vi "Stim_control_v17.vi"() -> ()   [LabVIEW 2010]
doc: "Use this template to measure or generate signals using the DAQ Assistant Express VI and NI-DAQmx. Double click the DAQ Assistant Express VI to launch a configuration wizard which steps you through configuring a measurement or generation.\n\nNote: You must have an NI-DAQmx compatible device installed to use this Express VI. Refer to the DAQ Quick Start Guide for NI-DAQ 7.0 for a list of compatible devices."
uses:
  <vilib>/Analysis/3filter.llb/Filter Passband Type.ctl
  <vilib>/DAQmx/write.llb/DAQmx Write (Digital Bool 1Line 1Point).vi
  <vilib>/DAQmx/write.llb/DAQmx Write (Analog 1D DBL 1Chan NSamp).vi
  <vilib>/DAQmx/read.llb/DAQmx Read (Analog 2D I16 NChan NSamp).vi
  <vilib>/daqmx/miscellaneous.llb/DAQmx Fill In Error Info.vi
  <vilib>/Utility/file.llb/Write To Spreadsheet File (DBL).vi
  <vilib>/DAQmx/create/channels.llb/DAQmx Create Channel (DO-Digital Output).vi
  <vilib>/DAQmx/create/channels.llb/DAQmx Create Channel (AO-Voltage-Basic).vi
  <vilib>/DAQmx/configure/timing.llb/DAQmx Timing (Sample Clock).vi
  <vilib>/DAQmx/configure/trigger.llb/DAQmx Start Trigger (Digital Edge).vi
  <vilib>/DAQmx/create/channels.llb/DAQmx Create Channel (AI-Voltage-Basic).vi
  Program Files/National Instruments/LabVIEW 2010/resource/objmgr/daqmx.rc
  <vilib>/Analysis/NI_AALBase.lvlib
  <vilib>/ptbypt/NI_PtbyPt.lvlib
panel:
  in  "ms to check for trigger":u32=5
  out "within file Datapoint number":u32
  out "Datapoint number":u32
  out "Detect On":bool
  out "Packet Size":i32
  in  "Stims before saving new file":dbl=200.0
  out "stimtrain_savename":path
  out "Stim rate":dbl
  out "Stim train loaded?":bool
  out "N Files":u32=1
  in  "Output Data Root":path=path "C:/DATA/gr15lb165"
  out "Current File":path
  in  "Bird Name":string="gr15lb165_250uA_2pulses"
  in  "File Open?":bool
  out "Outfile RefNum":refnum<file>
  out "Catch?":bool
  out "stim train number":u32
  out "Reset Trig Error 2":errorcluster
  in  "Manual Trigger":bool
  in  "calibration On?":bool
  out "AI Error":errorcluster
  in  "Data Before Trig(s)":dbl=2.0 format="%.2f"
  out "Buffer Size":i32
  in  "Analog Input Config":T1={"AI Channels"="Dev1/ai0,Dev1/ai15", "Scan Rate(kHz)"=32.0, "Min Voltage"=-10.0, "Max Voltage"=10.0, "Chan Name"="AI"} {"Scan Rate(kHz)" format="%.2f"}
  out "AO Error":errorcluster
  out "Reset Trig Error1":errorcluster
  out "AO Started?":bool
  out "stim train":dbl[](array[numeric])
  in  "Trig Refac(s)":dbl=0.05 format="%.3f"
  out "Playback Length":dbl format="%#_4g"
  out "Actual AO Rate":sgl format="%#.15f"
  out "AO Nwrtn":u32
  out "task out":refnum<k21>
  in  "DIO Trigger Pin":tag="Dev1/port0/line0"
  out "DOtask":refnum<k21>
  in  "Cal pressure":dbl
  in  "Cal pressure Voltage":dbl
  in  "Zero pressure Voltage":dbl
  out "Rates":enum16{"11025", "22050", "44100", "8000"}[](array[ring])
  in  "Analog Output Config":T2={"Min Voltage"=-10.0, "Max Voltage"=10.0, "Channels"="Dev1/ao0", "Chan Name"="AO", "Trigger Source"="/Dev1/PFI0"}
  out "stim patterns":T3(array[cluster]) {"stim pattern" format="%#_13g"}
  in  "directory path":path=path "C:/DATA/TTL_pulse_waves_for_STIM"
  out "Stim Rate":dbl[](array[numeric])
  out "last loop time":u32
  out "Loop time":u32
  out "AO readin":i16[](graph)
  out "Stim Pattern":dbl[](graph)
  out "stim count":i32
  in  "stim latency (ms)":u32=100
  out "previous point":dbl
  out "time of last trigger":u32
  in  "thresh":dbl=50000.0
  in  "offset control (ms)":dbl=400.0
  out "Pressure Waveform":dbl[](graph)
  in  "stop":bool
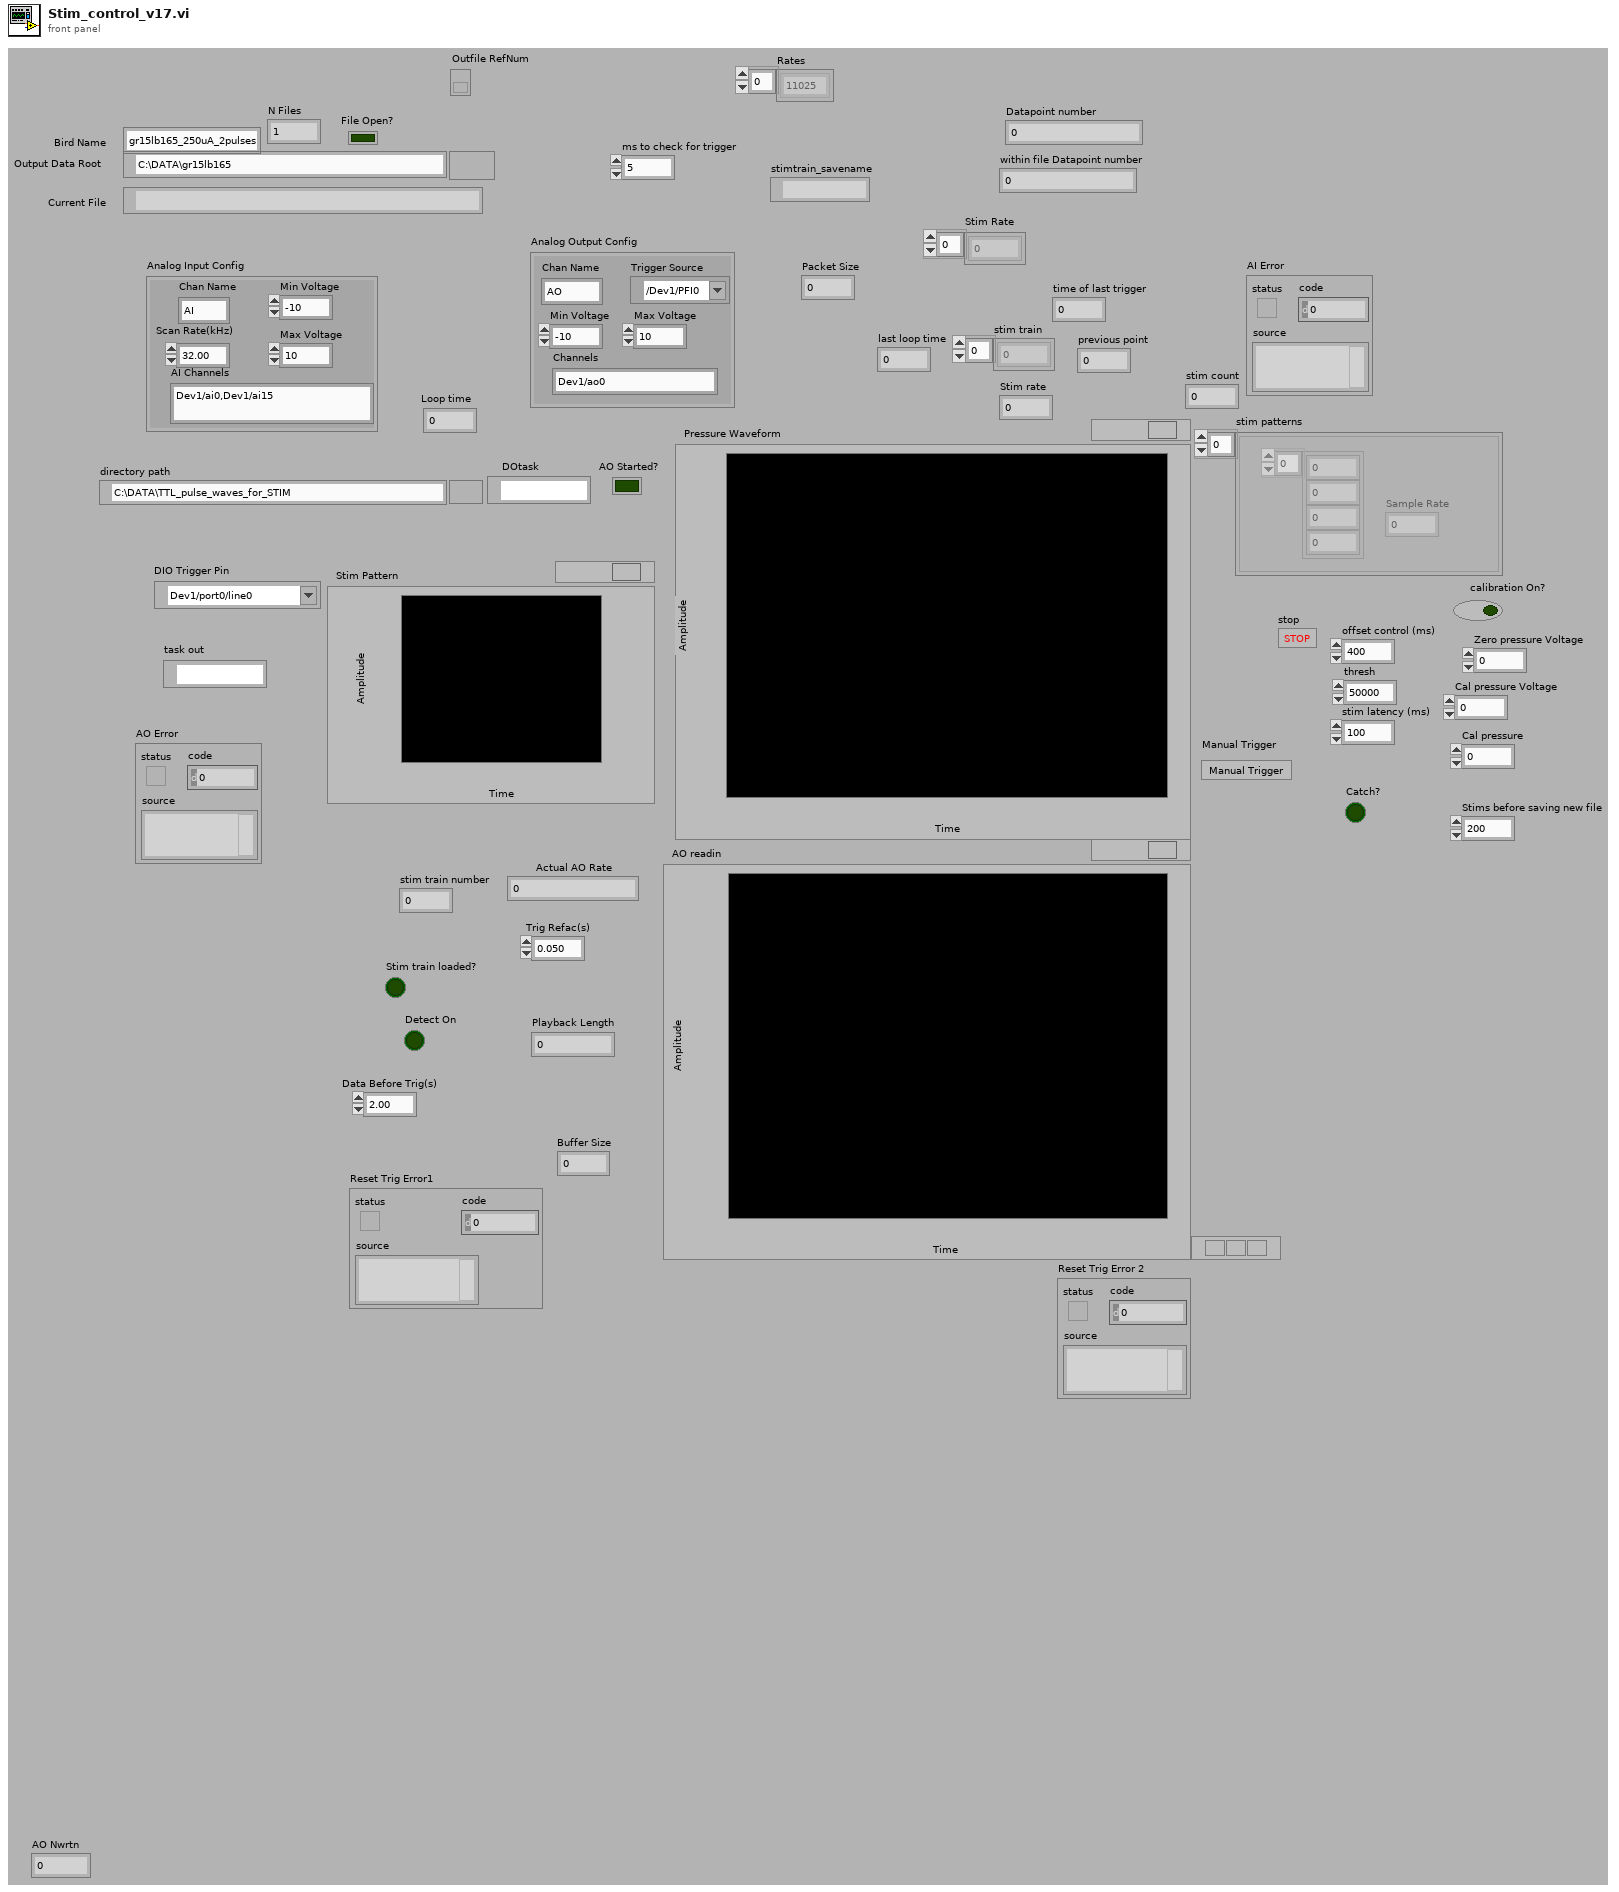
[diagram p1: front panel]
types:
  T1 = cluster{"AI Channels":string, "Scan Rate(kHz)":dbl, "Min Voltage":dbl, "Max Voltage":dbl, "Chan Name":string}
  T2 = cluster{"Min Voltage":dbl, "Max Voltage":dbl, "Channels":string, "Chan Name":string, "Trigger Source":tag}
  T3 = cluster{"stim pattern":dbl[], "Sample Rate":dbl}[]
  T4 = typedef "NI_AALBase.lvlib/Filter Passband Type.ctl" = enum32{"Lowpass", "Highpass", "Bandpass", "Bandstop"}
  T5 = typedef "Sound Format.ctl" = cluster{"sound quality":enum16{"mono", "stereo"}, "rate":enum16{"11025", "22050", "44100", "8000"}, "bits per sample":enum16{"8 bit", "16 bit"}}
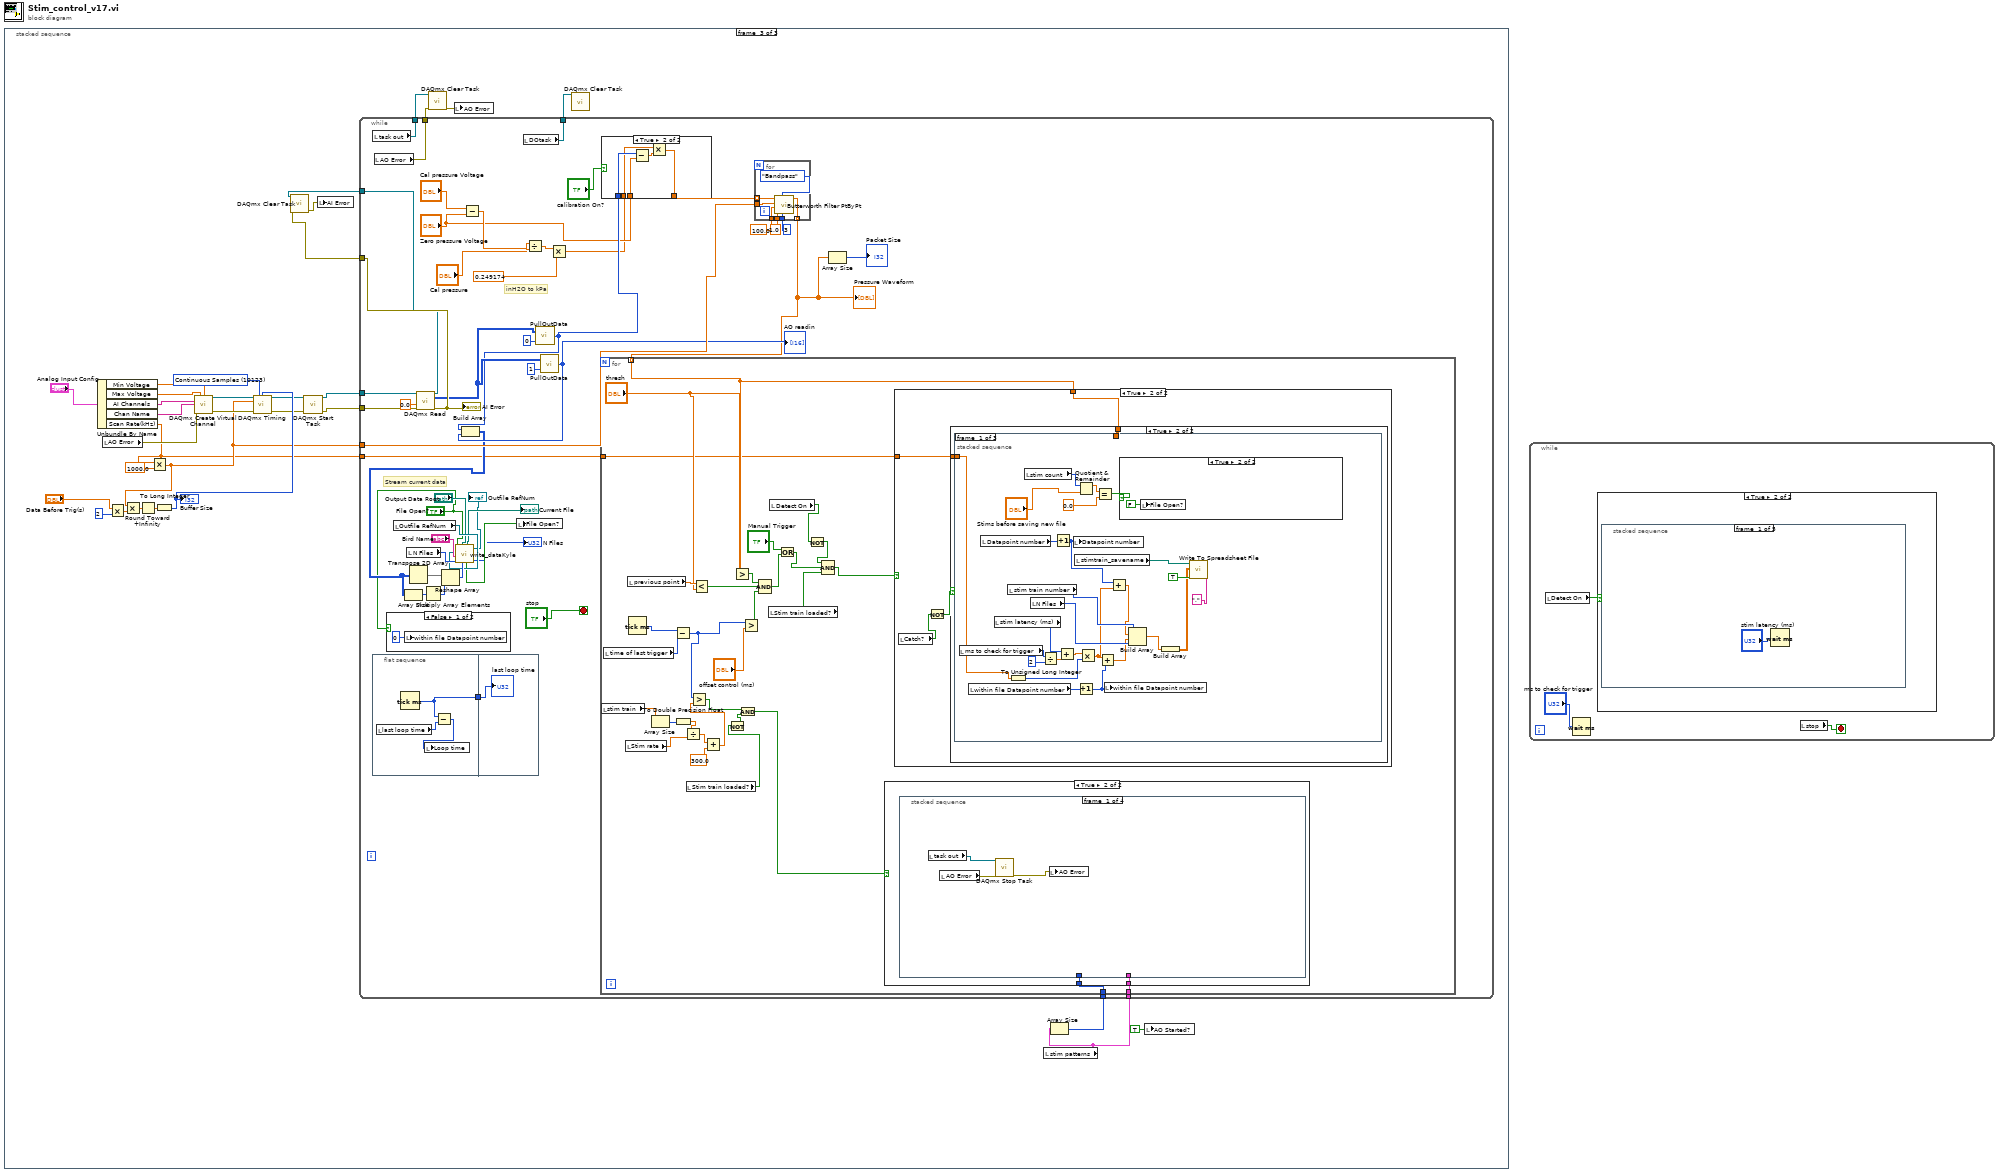
[diagram p0: block diagram]
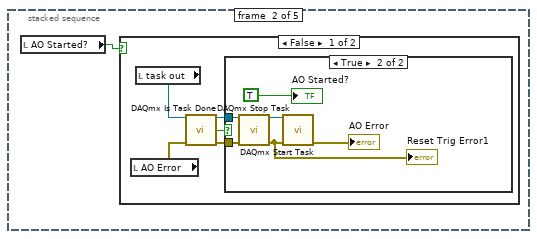
[diagram p3: hidden frame]
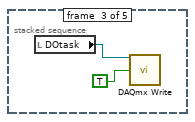
[diagram p6: hidden frame]
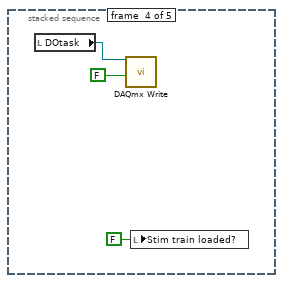
[diagram p7: hidden frame]
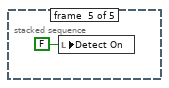
[diagram p8: hidden frame]
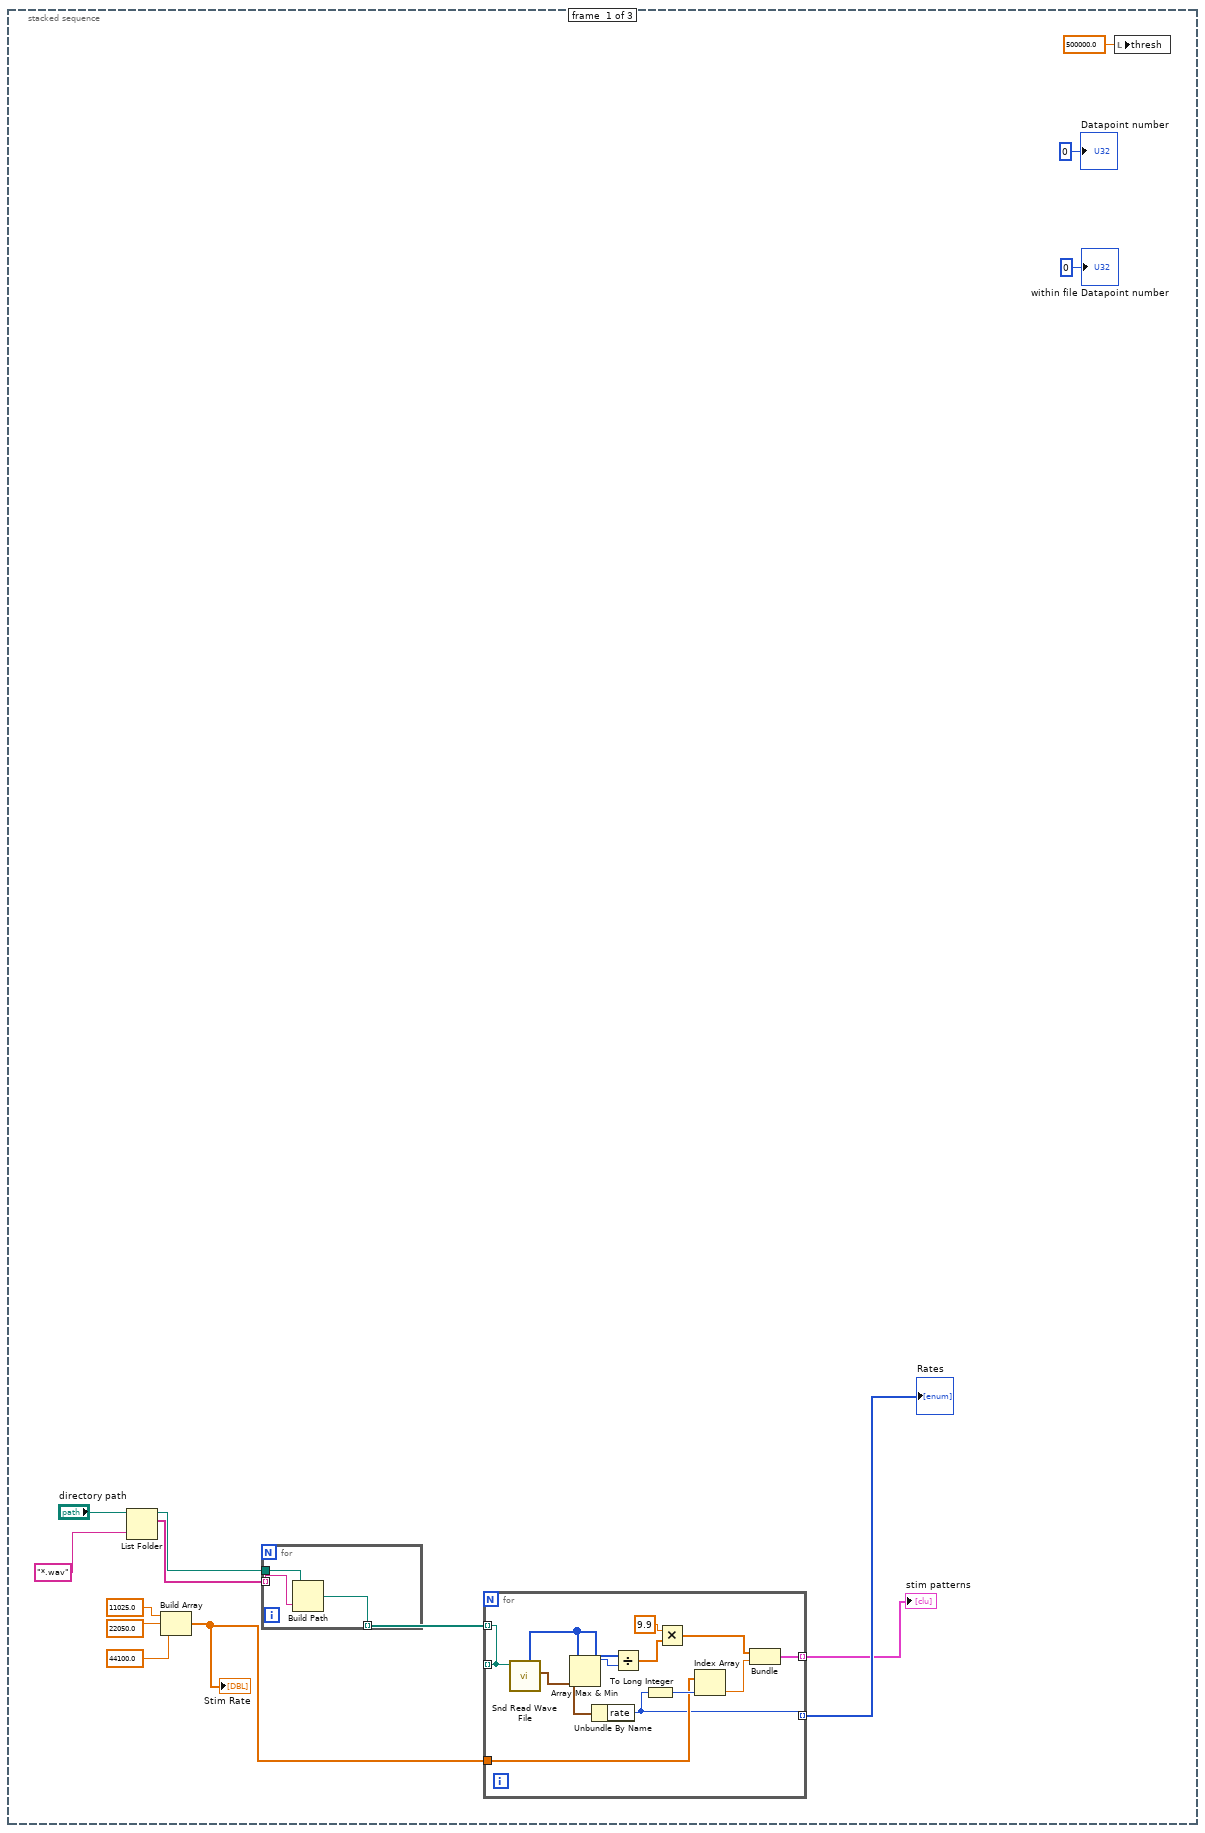
[diagram p9: hidden frame]
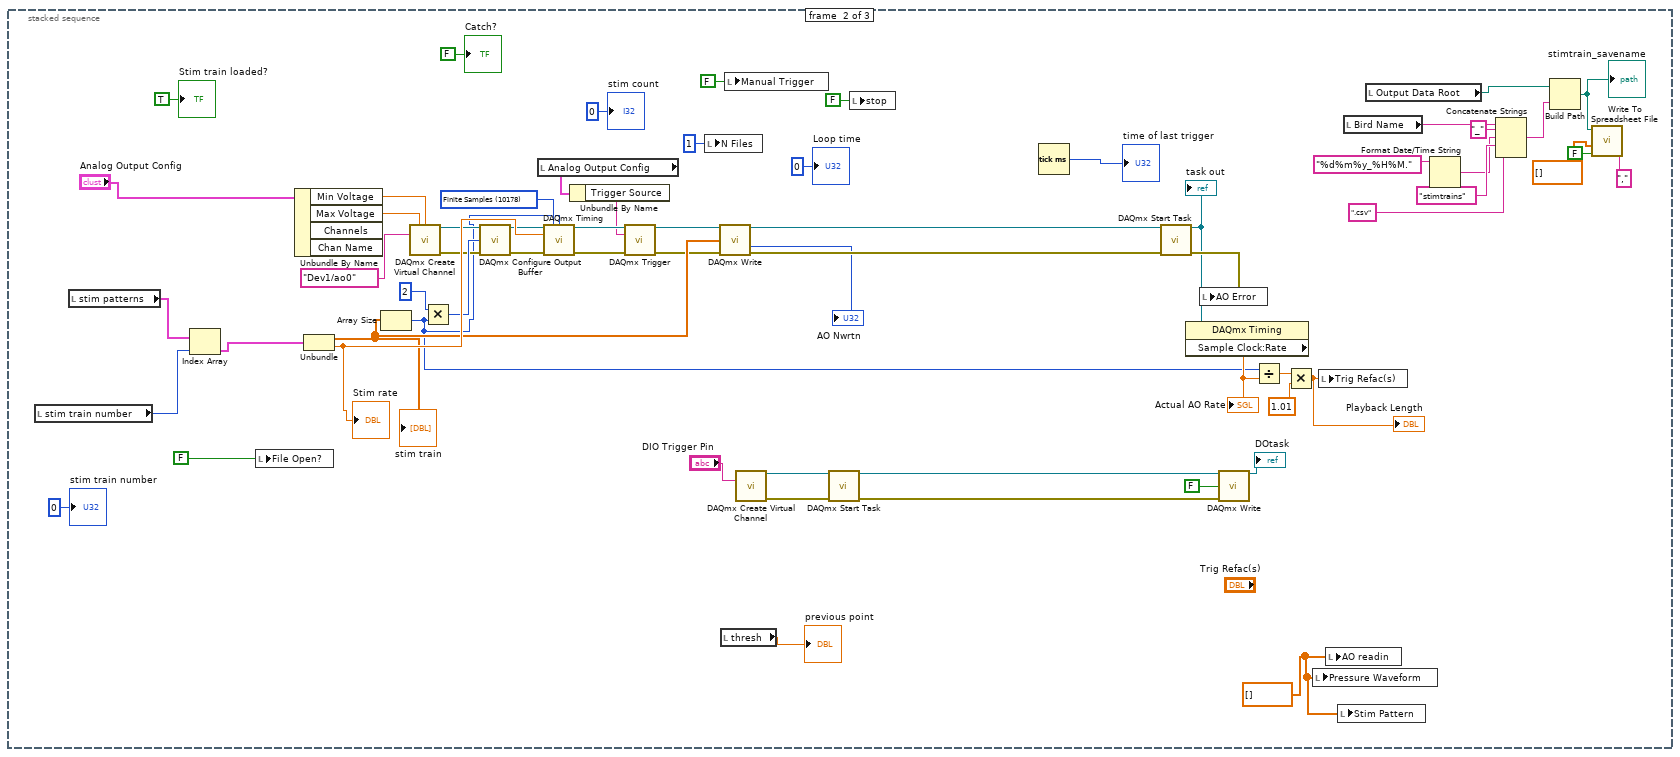
[diagram p10: hidden frame]
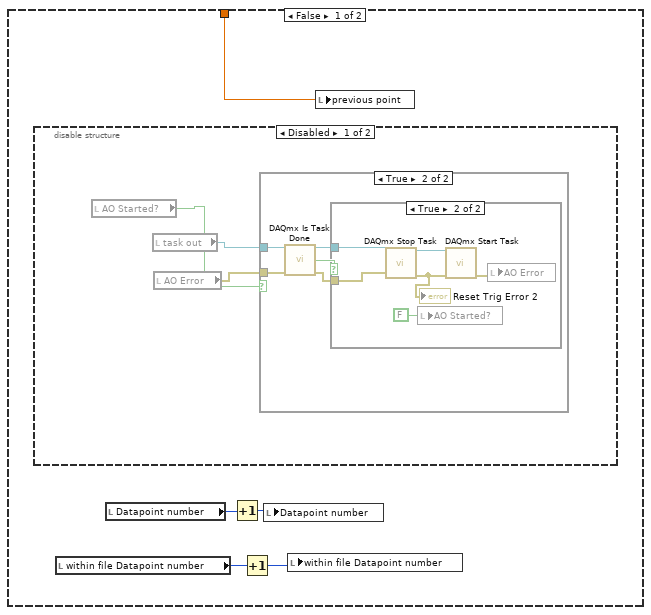
[diagram p13: hidden frame]
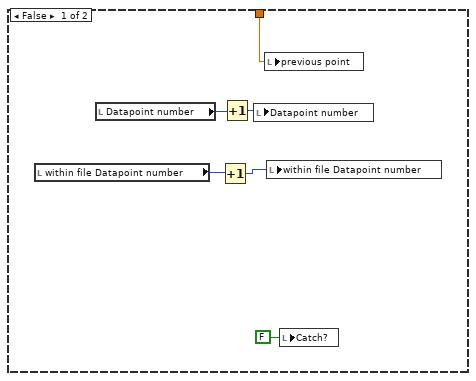
[diagram p17: hidden frame]
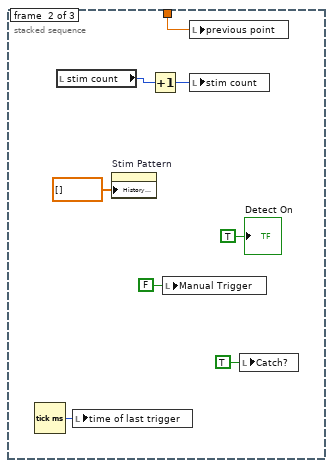
[diagram p19: hidden frame]
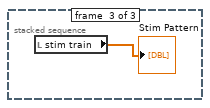
[diagram p20: hidden frame]
diagram:
  n1 = stacked-sequence {
    frame #0 {
      n2 = List Folder(path="directory path", pattern="*.wav") -> (path out=w10:path, filenames=w9:string[])  [unwired: 2 in, 2 out]
      n3 = Build Array(11025.0 ("element"), 22050.0 ("element"), 44100.0 ("element")) -> (w14:dbl[])
      "Stim Rate" <- w14
      n4 = for {
        tunnel: w9 -> [w27] mode=indexing
        tunnel: [w28] -> w13 mode=indexing
        tunnel: w10 -> [w29]
        n5 = Build Path(base path=w29, name or relative path=w27) -> (appended path=w28:path)
      }
      n6 = for {
        tunnel: [w15] -> _ mode=indexing
        tunnel: w14 -> [w24]
        tunnel: [w22] -> w11 mode=indexing
        tunnel: [w21] -> w12 mode=indexing
        tunnel: w13 -> [w15] mode=indexing
        n7 = call <vilib>:"Snd Read Wave File.vi"("wave file path"=w15) -> ("sound format"=w25:T5, "mono 16-bit"=w16:i16[])  [unwired: 4 in, 5 out]
        n8 = Array Max & Min(array=w16) -> (max value=w17:i16)  [unwired: 3 out]
        n9 = Unbundle By Name(w25) -> ("rate"=w21:enum16{"11025", "22050", "44100", "8000"})
        n10 = Divide(x=w16, y=w17) -> (x/y=w20:dbl[])
        n11 = To Long Integer(number=w21) -> (32bit integer=w26:i32)
        n12 = Multiply(x=9.9, y=w20) -> (x*y=w18:dbl[])
        n13 = Index Array(array=w24, index=w26) -> (element=w23:dbl)
        n14 = Bundle(w18, "element"=w23) -> (w22:cluster{dbl[], "element":dbl})  [unwired: 1 in]
      }
      "Rates" <- w12
      "stim patterns" <- w11
      n15 = local write "thresh"(500000.0 ("thresh")) -> ()
      "Datapoint number" <- 0 ("Datapoint number")
      "within file Datapoint number" <- 0 ("Datapoint number")
    }
    frame #1 {
      w43 = 10178 items=["Finite Samples"=10178, "Continuous Samples"=10123, "Hardware Timed Single Point"=12522] ("sample mode")
      w32 = dbl[] []
      n16 = local read "stim train number"() -> (w73:u32)
      n17 = local read "stim patterns"() -> (w64:T3)
      n18 = Index Array(array=w64, index=w73) -> (element=w65:cluster{"stim pattern":dbl[], "Sample Rate":dbl})
      n19 = local write "File Open?"(FALSE ("File Open?")) -> ()
      n20 = Unbundle By Name("Analog Output Config") -> ("Min Voltage"=w63:dbl, "Max Voltage"=w62:dbl)  [unwired: 2 out]
      n21 = Unbundle(w65) -> ("stim pattern"=w66:dbl[], "Sample Rate"=w76:dbl)
      "stim train" <- w66
      "Stim rate" <- w76
      n22 = Array Size(array=w66) -> (size(s)=w42:i32)
      n23 = call-poly <vilib>:"DAQmx Create Virtual Channel.vi"("maximum value"=w62, "minimum value"=w63, "physical channels"=tag "Dev1/ao0") -> ("task out"=w61:refnum<k21>, "error out"=w58:errorcluster)  [unwired: 11 in]
      n24 = Multiply(x=2, y=w42) -> (x*y=w59:i32)
      n25 = call <vilib>:"DAQmx Configure Output Buffer.vi"("task/channels in"=w61, "buffer size (in samples per channel)"=w59, "error in"=w58) -> ("task out"=w57:refnum<k21>, "error out"=w56:errorcluster)  [unwired: 11 in]
      n26 = local read "Analog Output Config"() -> (w54:T2)
      n27 = call-poly <vilib>:"DAQmx Timing.vi"("task/channels in"=w57, "sample mode"=w43, "samples per channel"=w42, "rate"=w76, "error in"=w56) -> ("task out"=w55:refnum<k21>, "error out"=w52:errorcluster)  [unwired: 9 in]
      n28 = Unbundle By Name(w54) -> ("Trigger Source"=w53:tag)
      n29 = call-poly <vilib>:"DAQmx Trigger.vi"("task/channels in"=w55, "source"=w53, "error in"=w52) -> ("task out"=w51:refnum<k21>, "error out"=w50:errorcluster)  [unwired: 11 in]
      n30 = local write "N Files"(i16 1 ("N Files")) -> ()
      n31 = call-poly <vilib>:"DAQmx Write.vi"("task/channels in"=w51, "data"=w66, "error in"=w50) -> ("task out"=w49:refnum<k21>, "number of samples written per channel"=→"AO Nwrtn":u32, "error out"=w48:errorcluster)  [unwired: 10 in]
      n32 = local read "thresh"() -> (→"previous point":dbl)
      n33 = local write "Manual Trigger"(FALSE ("Manual Trigger")) -> ()
      n34 = call-poly <vilib>:"DAQmx Create Virtual Channel.vi"("lines"="DIO Trigger Pin") -> ("task out"=w39:refnum<k21>, "error out"=w36:errorcluster)  [unwired: 13 in]
      n35 = call <vilib>:"DAQmx Start Task.vi"("task/channels in"=w39, "error in"=w36) -> ("task out"=w37:refnum<k21>, "error out"=w38:errorcluster)  [unwired: 12 in]
      n36 = local write "stop"(FALSE ("stop")) -> ()
      n37 = Tick Count (ms)() -> (millisecond timer value=→"time of last trigger":u32)
      n38 = call <vilib>:"DAQmx Start Task.vi"("task/channels in"=w49, "error in"=w48) -> ("task out"=w46:refnum<k21>, "error out"=w68:errorcluster)  [unwired: 12 in]
      "task out" <- w46
      n39 = property class="DAQmx Timing"(reference=w46) -> ("Sample Clock:Rate"=w45:dbl)  [unwired: 1 in, 2 out]
      "Actual AO Rate" <- w45
      n40 = local write "AO Error"(w68) -> ()
      n41 = call-poly <vilib>:"DAQmx Write.vi"("task/channels in"=w37, "data"=FALSE, "error in"=w38) -> ("task out"=→"DOtask":refnum<k21>)  [unwired: 10 in, 2 out]
      n42 = Divide(x=w42, y=w45) -> (x/y=w41:dbl)
      n43 = Multiply(x=w41, y=1.01) -> (x*y=w74:dbl)
      "Playback Length" <- w74
      n44 = local write "Pressure Waveform"(w32) -> ()
      n45 = local write "Trig Refac(s)"(w74) -> ()
      n46 = local write "AO readin"(w32) -> ()
      n47 = local write "Stim Pattern"(w32) -> ()
      n48 = local read "Bird Name"() -> (w79:string)
      n49 = local read "Output Data Root"() -> (w78:path)
      n50 = Format Date/Time String(time format string (%c)="%d%m%y_%H%M.") -> (date/time string=w82:string)  [unwired: 2 in]
      n51 = Concatenate Strings(w79, "_" ("string"), w82, "stimtrains" ("string"), ".csv" ("Substring")) -> (w85:string)
      n52 = Build Path(base path=w78, name or relative path=w85) -> (appended path=w86:path)
      "stimtrain_savename" <- w86
      n53 = call-poly <vilib>:"Write To Spreadsheet File.vi"("delimiter (\\t)"="," ("delimiter (\\t)"), "append to file? (new file:F)"=FALSE, "1D data"=dbl[] [], "file path (dialog if empty)"=w86) -> ()  [unwired: 4 in, 1 out]
      "stim count" <- 0 ("stim count")
      "stim train number" <- i16 0 ("stim train number")
      "Catch?" <- FALSE ("Catch?")
      "Stim train loaded?" <- TRUE ("Stim train loaded?")
      "Loop time" <- u32 0 ("Loop time")
    }
    frame #2 {
      w109 = 10123 items=["Finite Samples"=10178, "Continuous Samples"=10123, "Hardware Timed Single Point"=12522] ("sample mode")
      n54 = Unbundle By Name("Analog Input Config") -> ("Min Voltage"=w118:dbl, "Max Voltage"=w119:dbl, "AI Channels"=w121:string, "Chan Name"=w120:string, "Scan Rate(kHz)"=w93:dbl)
      n55 = local read "AO Error"() -> (w94:errorcluster)
      n56 = Multiply(x="Data Before Trig(s)", y=2) -> (x*y=w112:dbl)
      n57 = Multiply(x=w93, y=1000.0) -> (x*y=w100:dbl)
      n58 = Multiply(x=w100, y=w112) -> (x*y=w113:dbl)
      n59 = Round Toward +Infinity(x=w113) -> (ceil(x): smallest int >= x=w114:dbl)
      n60 = To Long Integer(number=w114) -> (32bit integer=w110:i32)
      "Buffer Size" <- w110
      n61 = call-poly <vilib>:"DAQmx Create Virtual Channel.vi"("maximum value"=w119, "minimum value"=w118, "physical channels"=w121, "name to assign"=w120, "error in"=w94) -> ("task out"=w117:refnum<k21>, "error out"=w116:errorcluster)  [unwired: 9 in]
      n62 = call-poly <vilib>:"DAQmx Timing.vi"("task/channels in"=w117, "sample mode"=w109, "samples per channel"=w110, "rate"=w100, "error in"=w116) -> ("task out"=w108:refnum<k21>, "error out"=w107:errorcluster)  [unwired: 9 in]
      n63 = call <vilib>:"DAQmx Start Task.vi"("task/channels in"=w108, "error in"=w107) -> ("task out"=w106:refnum<k21>, "error out"=w105:errorcluster)  [unwired: 12 in]
      n64 = local read "stim patterns"() -> (w123:T3)
      n65 = Array Size(array=w123) -> (size(s)=w124:i32)
      n66 = while {
        tunnel: w124 -> [w170]
        tunnel: w123 -> [w169]
        tunnel: w106 -> [w168]
        tunnel: w105 -> [w167]
        tunnel: [w165] -> w104
        tunnel: [w164] -> w102
        tunnel: w100 -> [w160]
        tunnel: [w148] -> w98
        tunnel: [w147] -> w97
        tunnel: [w146] -> w95
        tunnel: w93 -> [w125]
        stop <- "stop" stop-if-true
        # "Stream current data"
        # "inH2O to kPa"
        n67 = local read "task out"() -> (w148:refnum<k21>)
        n68 = flat-sequence {
          tunnel: [w175] -> w127
          tunnel: w127 -> [w176]
          frame #0 {
            n69 = local read "last loop time"() -> (w174:u32)
            n70 = Tick Count (ms)() -> (millisecond timer value=w175:u32)
            n71 = Subtract(x=w175, y=w174) -> (x-y=w173:u32)
            n72 = local write "Loop time"(w173) -> ()
          }
          frame #1 {
            "last loop time" <- w176
          }
        }
        n73 = local read "AO Error"() -> (w147:errorcluster)
        n74 = case shown="False" "File Open?" {
          frame False {
            n75 = local write "within file Datapoint number"(u32 0 ("within file Datapoint number")) -> ()
          }
          frame True {
          }
        }
        n76 = local read "Outfile RefNum"() -> (w133:refnum<file>)
        n77 = local read "N Files"() -> (w134:u32)
        n78 = call-poly <vilib>:"DAQmx Read.vi"("task/channels in"=w168, "timeout"=0.0, "error in"=w167) -> ("task out"=w164:refnum<k21>, "data"=w159:i16[][], "error out"=w165:errorcluster)  [unwired: 10 in]
        "AI Error" <- w165
        n79 = Subtract(x="Cal pressure Voltage", y="Zero pressure Voltage") -> (x-y=w156:dbl)
        n80 = local read "DOtask"() -> (w146:refnum<k21>)
        n81 = Divide(x="Cal pressure", y=w156) -> (x/y=w153:dbl)
        n82 = call "PullOutData.vi"("WhichInd"=0, "InputArray"=w159) -> ("OutVec"=w158:i16[])
        n83 = call "PullOutData.vi"("WhichInd"=1, "InputArray"=w159) -> ("OutVec"=w157:i16[])
        "AO readin" <- w157
        n84 = Build Array(w158, w157) -> (w149:i16[][])
        n85 = Array Size(array=w149) -> (size(s)=w139:i32[])
        n86 = Transpose 2D Array(2D array=w149) -> (transposed array=w138:i16[][])
        n87 = Multiply Array Elements(1:w139) -> (0:w137:i32)
        n88 = Reshape Array(w138, w137) -> (w135:i16[])
        n89 = call "write_dataKyle.vi"("Root Path"="Output Data Root", "File Open In"="File Open?", "RefNum In"=w133, "Data"=w135, "Bird Name"="Bird Name", "N Files In"=w134) -> ("RefNum Out"=→"Outfile RefNum":refnum<file>, "Output File Path"=→"Current File":path, "N Files Out"=→"N Files":i16, "File Open Out"=w129:bool)  [unwired: 1 in]
        n90 = local write "File Open?"(w129) -> ()
        n91 = Multiply(x=w153, y=0.249174) -> (x*y=w150:dbl)
        n92 = case shown="True" "calibration On?" {
          tunnel: w158 -> [w184 w189]
          tunnel: "Zero pressure Voltage" -> [_ w188]
          tunnel: w150 -> [_ w186]
          tunnel: [w184 w185] -> w140
          frame False {
          }
          frame True {
            n93 = Subtract(x=w189, y=w188) -> (x-y=w187:dbl[])
            n94 = Multiply(x=w186, y=w187) -> (x*y=w185:dbl[])
          }
        }
        n95 = for {
          tunnel: w140 -> [w182] mode=indexing
          tunnel: [w181] -> w141 mode=indexing
          tunnel: 100.0 ("high cutoff freq: fh") -> [w180]
          tunnel: 1.0 ("low cutoff freq: fl") -> [w179]
          tunnel: w160 -> [w178]
          tunnel: 3 ("order") -> [w177]
          n96 = call <vilib>:"Butterworth Filter PtByPt.vi"("order"=w177, "filter type"=Filter_Passband_Type."Bandpass", "low cutoff freq: fl"=w179, "high cutoff freq: fh"=w180, "sampling freq: fs"=w178, "x"=w182) -> ("Filtered x"=w181:dbl)  [unwired: 3 in, 1 out]
        }
        "Pressure Waveform" <- w141
        n97 = for {
          tunnel: w141 -> [w215] mode=indexing
          tunnel: w170 -> [w200]
          tunnel: w169 -> [w199]
          tunnel: w125 -> [w190]
          n98 = local read "stim train"() -> (w208:dbl[])
          n99 = local read "time of last trigger"() -> (w217:u32)
          n100 = local read "Stim rate"() -> (w193:dbl)
          n101 = local read "previous point"() -> (w214:dbl)
          n102 = Tick Count (ms)() -> (millisecond timer value=w218:u32)
          n103 = Array Size(array=w208) -> (size(s)=w195:i32)
          n104 = Subtract(x=w218, y=w217) -> (x-y=w209:u32)
          n105 = To Double Precision Float(number=w195) -> (double precision float=w194:dbl)
          n106 = Divide(x=w194, y=w193) -> (x/y=w207:dbl)
          n107 = local read "Stim train loaded?"() -> (w202:bool)
          n108 = Less?(x=w214, y="thresh") -> (x < y?=w212:bool)
          n109 = Add(x=w207, y=300.0) -> (x+y=w205:dbl)
          n110 = Greater?(x=w209, y=w205) -> (0:w204:bool)
          n111 = Not(x=w202) -> (.not. x?=w203:bool)
          n112 = Greater?(x=w215, y="thresh") -> (0:w220:bool)
          n113 = And(x=w204, y=w203) -> (x .and. y?=w201:bool)
          n114 = Greater?(x=w209, y="offset control (ms)") -> (0:w216:bool)
          n115 = Compound Arithmetic op=AND(w220, w212, w216) -> (w210:bool)
          n116 = local read "Stim train loaded?"() -> (w196:bool)
          n117 = local read "Detect On"() -> (w191:bool)
          n118 = Or(x="Manual Trigger", y=w210) -> (x .or. y?=w197:bool)
          n119 = Not(x=w191) -> (.not. x?=w192:bool)
          n120 = Compound Arithmetic op=AND(w192, w197, w196) -> (w198:bool)
          n121 = case shown="True" w201 {
            tunnel: w200 -> [_ w289]
            tunnel: w199 -> [_ w288]
            frame False {
            }
            frame True {
              n122 = stacked-sequence {
                tunnel: w289 -> [_ w294 _ _]
                tunnel: w288 -> [_ w293 _ _]
                frame #0 {
                  n123 = local read "task out"() -> (w291:refnum<k21>)
                  n124 = local read "AO Error"() -> (w290:errorcluster)
                  n125 = call <vilib>:"DAQmx Stop Task.vi"("task/channels in"=w291, "error in"=w290) -> ("error out"=w292:errorcluster)  [unwired: 12 in, 1 out]
                  n126 = local write "AO Error"(w292) -> ()
                }
                frame #1 {
                  n127 = local read "stim count"() -> (w298:i32)
                  n128 = Quotient & Remainder(x=w298, y=w294) -> (x-y*floor(x/y)=w297:i32)  [unwired: 1 out]
                  n129 = Index Array(array=w293, index=w297) -> (element=w296:cluster{"stim pattern":dbl[], "Sample Rate":dbl})
                  n130 = local write "stim train number"(w297) -> ()
                  n131 = Unbundle(w296) -> ("stim pattern"=w295:dbl[])  [unwired: 1 out]
                  n132 = local write "stim train"(w295) -> ()
                }
                frame #2 {
                  w313 = 10178 items=["Finite Samples"=10178, "Continuous Samples"=10123, "Hardware Timed Single Point"=12522] ("sample mode")
                  n133 = local read "stim train"() -> (w310:dbl[])
                  n134 = local read "AO Error"() -> (w299:errorcluster)
                  n135 = local read "task out"() -> (w300:refnum<k21>)
                  n136 = Array Size(array=w310) -> (size(s)=w303:i32)
                  n137 = Multiply(x=2, y=w303) -> (x*y=w314:i32)
                  n138 = local read "Stim rate"() -> (w301:dbl)
                  n139 = local read "Analog Output Config"() -> (w312:T2)
                  n140 = call <vilib>:"DAQmx Configure Output Buffer.vi"("task/channels in"=w300, "buffer size (in samples per channel)"=w314, "error in"=w299) -> ("task out"=w323:refnum<k21>, "error out"=w316:errorcluster)  [unwired: 11 in]
                  n141 = call-poly <vilib>:"DAQmx Timing.vi"("task/channels in"=w323, "sample mode"=w313, "samples per channel"=w303, "rate"=w301, "error in"=w316) -> ("task out"=w322:refnum<k21>, "error out"=w317:errorcluster)  [unwired: 9 in]
                  n142 = Unbundle By Name(w312) -> ("Trigger Source"=w311:tag)
                  n143 = call-poly <vilib>:"DAQmx Trigger.vi"("task/channels in"=w322, "source"=w311, "error in"=w317) -> ("task out"=w321:refnum<k21>, "error out"=w318:errorcluster)  [unwired: 11 in]
                  n144 = call-poly <vilib>:"DAQmx Write.vi"("task/channels in"=w321, "data"=w310, "error in"=w318) -> ("task out"=w320:refnum<k21>, "number of samples written per channel"=w309:u32, "error out"=w319:errorcluster)  [unwired: 10 in]
                  n145 = local write "AO Nwrtn"(w309) -> ()
                  n146 = call <vilib>:"DAQmx Start Task.vi"("task/channels in"=w320, "error in"=w319) -> ("task out"=w302:refnum<k21>, "error out"=w308:errorcluster)  [unwired: 12 in]
                  n147 = property class="DAQmx Timing"(reference=w302) -> ("Sample Clock:Rate"=w305:dbl)  [unwired: 1 in, 2 out]
                  n148 = local write "Actual AO Rate"(w305) -> ()
                  n149 = Divide(x=w303, y=w305) -> (x/y=w307:dbl)
                  n150 = Multiply(x=w307, y=1.01) -> (x*y=w304:dbl)
                  n151 = local write "Trig Refac(s)"(w304) -> ()
                  n152 = local write "Playback Length"(w304) -> ()
                  n153 = local write "task out"(w302) -> ()
                  n154 = local write "AO Error"(w308) -> ()
                }
                frame #3 {
                  n155 = local write "Stim train loaded?"(TRUE ("Stim train loaded?")) -> ()
                }
              }
            }
          }
          n156 = case shown="True" w198 {
            tunnel: w215 -> [w225 w243]
            tunnel: w190 -> [_ w240]
            frame False {
              n157 = disable-structure shown="Disabled" {
                frame Disabled {
                  n158 = local read "AO Started?"() -> (w226:bool)
                  n159 = local read "task out"() -> (w228:refnum<k21>)
                  n160 = local read "AO Error"() -> (w227:errorcluster)
                  n161 = case shown="True" w226 {
                    tunnel: w228 -> [_ w233]
                    tunnel: w227 -> [_ w232]
                    frame False {
                    }
                    frame True {
                      n162 = call <vilib>:"DAQmx Is Task Done.vi"("task/channels in"=w233, "error in"=w232) -> ("task out"=w230:refnum<k21>, "task done?"=w231:bool, "error out"=w229:errorcluster)  [unwired: 11 in]
                      n163 = case shown="True" w231 {
                        tunnel: w230 -> [_ w239]
                        tunnel: w229 -> [_ w237]
                        frame False {
                        }
                        frame True {
                          n164 = call <vilib>:"DAQmx Stop Task.vi"("task/channels in"=w239, "error in"=w237) -> ("task out"=w238:refnum<k21>, "error out"=w234:errorcluster)  [unwired: 12 in]
                          "Reset Trig Error 2" <- w234
                          n165 = local write "AO Started?"(FALSE ("AO Started?")) -> ()
                          n166 = call <vilib>:"DAQmx Start Task.vi"("task/channels in"=w238, "error in"=w234) -> ("error out"=w236:errorcluster)  [unwired: 12 in, 1 out]
                          n167 = local write "AO Error"(w236) -> ()
                        }
                      }
                    }
                  }
                }
                frame Enabled {
                }
              }
              n168 = local read "within file Datapoint number"() -> (w222:u32)
              n169 = local read "Datapoint number"() -> (w223:u32)
              n170 = Increment(x=w223) -> (x+1=w224:u32)
              n171 = Increment(x=w222) -> (x+1=w221:u32)
              n172 = local write "Datapoint number"(w224) -> ()
              n173 = local write "within file Datapoint number"(w221) -> ()
              n174 = local write "previous point"(w225) -> ()
            }
            frame True {
              n175 = local read "Catch?"() -> (w242:bool)
              n176 = Not(x=w242) -> (.not. x?=w241:bool)
              n177 = case shown="True" w241 {
                tunnel: w243 -> [w248 w251]
                tunnel: w240 -> [_ w250]
                frame False {
                  n178 = local read "within file Datapoint number"() -> (w245:u32)
                  n179 = local read "Datapoint number"() -> (w246:u32)
                  n180 = Increment(x=w245) -> (x+1=w244:u32)
                  n181 = Increment(x=w246) -> (x+1=w247:u32)
                  n182 = local write "Datapoint number"(w247) -> ()
                  n183 = local write "previous point"(w248) -> ()
                  n184 = local write "within file Datapoint number"(w244) -> ()
                  n185 = local write "Catch?"(FALSE ("Catch?")) -> ()
                }
                frame True {
                  n186 = stacked-sequence {
                    tunnel: w251 -> [_ w283 _]
                    tunnel: w250 -> [w261 _ _]
                    frame #0 {
                      n187 = local read "ms to check for trigger"() -> (w257:u32)
                      n188 = local read "within file Datapoint number"() -> (w264:u32)
                      n189 = local read "Datapoint number"() -> (w269:u32)
                      n190 = local read "stim latency (ms)"() -> (w259:u32)
                      n191 = local read "stim train number"() -> (w266:u32)
                      n192 = To Unsigned Long Integer(number=w261) -> (unsigned 32bit integer=w260:u32)
                      n193 = local read "stim count"() -> (w271:i32)
                      n194 = local read "N Files"() -> (w265:u32)
                      n195 = Divide(x=w257, y=u32 2) -> (x/y=w256:dbl)
                      n196 = Increment(x=w269) -> (x+1=w254:u32)
                      n197 = Add(x=w259, y=w256) -> (x+y=w258:dbl)
                      n198 = local write "Datapoint number"(w254) -> ()
                      n199 = local read "stimtrain_savename"() -> (w277:path)
                      n200 = Quotient & Remainder(x=w271, y="Stims before saving new file") -> (x-y*floor(x/y)=w273:dbl)  [unwired: 1 out]
                      n201 = Increment(x=w264) -> (x+1=w263:u32)
                      n202 = Multiply(x=w258, y=w260) -> (x*y=w252:dbl)
                      n203 = Equal?(x=w273, y=0.0) -> (x = y?=w274:bool)
                      n204 = Add(x=w252, y=w263) -> (x+y=w262:dbl)
                      n205 = local write "within file Datapoint number"(w263) -> ()
                      n206 = Add(x=w254, y=w252) -> (x+y=w253:dbl)
                      n207 = case shown="True" w274 {
                        frame False {
                        }
                        frame True {
                          n208 = local write "File Open?"(FALSE ("File Open?")) -> ()
                        }
                      }
                      n209 = Build Array(w266, w253, w262, w265) -> (w268:dbl[])
                      n210 = Build Array(w268) -> (w267:dbl[][])
                      n211 = call-poly <vilib>:"Write To Spreadsheet File.vi"("delimiter (\\t)"="," ("delimiter (\\t)"), "append to file? (new file:F)"=TRUE, "2D data"=w267, "file path (dialog if empty)"=w277) -> ()  [unwired: 4 in, 1 out]
                    }
                    frame #1 {
                      n212 = Tick Count (ms)() -> (millisecond timer value=w286:u32)
                      n213 = local read "stim count"() -> (w284:i32)
                      n214 = local write "time of last trigger"(w286) -> ()
                      n215 = property on="Stim Pattern" class="WFChart (strict)"("History Data"=dbl[] []) -> ()  [unwired: 2 in, 2 out]
                      n216 = Increment(x=w284) -> (x+1=w285:i32)
                      n217 = local write "Manual Trigger"(FALSE ("Manual Trigger")) -> ()
                      n218 = local write "previous point"(w283) -> ()
                      n219 = local write "stim count"(w285) -> ()
                      n220 = local write "Catch?"(TRUE ("Catch?")) -> ()
                      "Detect On" <- TRUE ("Detect On")
                    }
                    frame #2 {
                      n221 = local read "stim train"() -> (→"Stim Pattern":dbl[])
                    }
                  }
                }
              }
            }
          }
        }
        n222 = Array Size(array=w141) -> (size(s)=→"Packet Size":i32)
      }
      n223 = call <vilib>:"DAQmx Clear Task.vi"("task in"=w102, "error in"=w104) -> ("error out"=w103:errorcluster)  [unwired: 13 in]
      n224 = local write "AI Error"(w103) -> ()
      n225 = call <vilib>:"DAQmx Clear Task.vi"("task in"=w98, "error in"=w97) -> ("error out"=w96:errorcluster)  [unwired: 13 in]
      n226 = local write "AO Error"(w96) -> ()
      n227 = call <vilib>:"DAQmx Clear Task.vi"("task in"=w95) -> ()  [unwired: 14 in, 1 out]
      n228 = local write "AO Started?"(TRUE ("AO Started?")) -> ()
    }
  }
  n229 = while {
    stop <- w327 stop-if-true
    n230 = local read "Detect On"() -> (w326:bool)
    n231 = Wait (ms)(milliseconds to wait="ms to check for trigger") -> ()  [unwired: 1 out]
    n232 = case shown="True" w326 {
      frame False {
      }
      frame True {
        n233 = stacked-sequence {
          frame #0 {
            n234 = Wait (ms)(milliseconds to wait="stim latency (ms)") -> ()  [unwired: 1 out]
          }
          frame #1 {
            n235 = local read "AO Started?"() -> (w329:bool)
            n236 = case shown="False" w329 {
              frame False {
                n237 = local read "AO Error"() -> (w334:errorcluster)
                n238 = local read "task out"() -> (w333:refnum<k21>)
                n239 = call <vilib>:"DAQmx Is Task Done.vi"("task/channels in"=w333, "error in"=w334) -> ("task out"=w332:refnum<k21>, "task done?"=w330:bool, "error out"=w331:errorcluster)  [unwired: 11 in]
                n240 = case shown="True" w330 {
                  tunnel: w332 -> [_ w337]
                  tunnel: w331 -> [_ w336]
                  frame False {
                  }
                  frame True {
                    n241 = call <vilib>:"DAQmx Stop Task.vi"("task/channels in"=w337, "error in"=w336) -> ("task out"=w340:refnum<k21>, "error out"=w338:errorcluster)  [unwired: 12 in]
                    "Reset Trig Error1" <- w338
                    n242 = call <vilib>:"DAQmx Start Task.vi"("task/channels in"=w340, "error in"=w338) -> ("error out"=→"AO Error":errorcluster)  [unwired: 12 in, 1 out]
                    "AO Started?" <- TRUE ("Tirg Last It")
                  }
                }
              }
              frame True {
              }
            }
          }
          frame #2 {
            n243 = local read "DOtask"() -> (w342:refnum<k21>)
            n244 = call-poly <vilib>:"DAQmx Write.vi"("task/channels in"=w342, "data"=TRUE) -> ()  [unwired: 11 in, 3 out]
          }
          frame #3 {
            n245 = local read "DOtask"() -> (w343:refnum<k21>)
            n246 = call-poly <vilib>:"DAQmx Write.vi"("task/channels in"=w343, "data"=FALSE) -> ()  [unwired: 11 in, 3 out]
            n247 = local write "Stim train loaded?"(FALSE ("Stim train loaded?")) -> ()
          }
          frame #4 {
            n248 = local write "Detect On"(FALSE ("Detect On")) -> ()
          }
        }
      }
    }
    n249 = local read "stop"() -> (w327:bool)
  }
